vi "Post-Install Custom Action.vi"(10 "Variant":variant) -> (0 "error out":errorcluster)   [LabVIEW 2020]
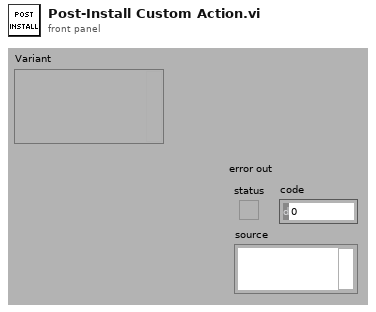
[diagram p1: front panel]
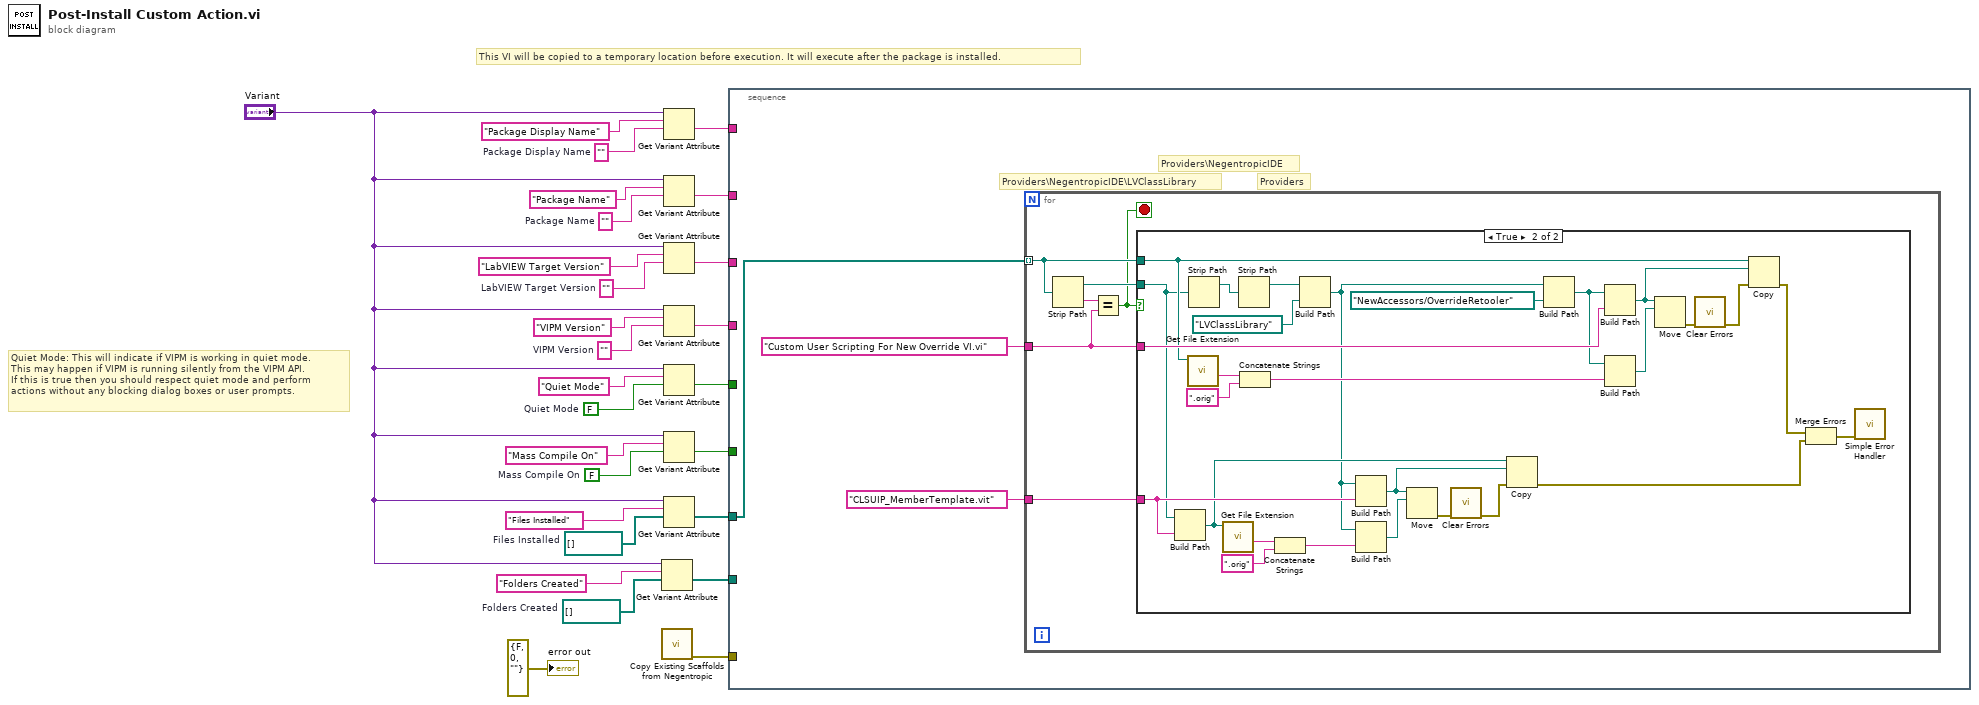
[diagram p0: block diagram]
diagram:
  w2 = path[] []  # Folders Created
  w3 = path[] []  # Files Installed
  w9 = FALSE  # Mass Compile On
  w10 = ""  # Package Display Name
  w17 = FALSE  # Quiet Mode
  w20 = ""  # VIPM Version
  w22 = ""  # LabVIEW Target Version
  w24 = ""  # Package Name
  # "Quiet Mode: This will indicate if VIPM is working in quiet mode.\nThis may happen if VIPM is running silently from the VIPM API.\nIf this is true then you should respect quiet mode and perform\nactions without any blocking dialog boxes or user prompts."
  # "This VI will be copied to a temporary location before execution. It will execute after the package is installed."
  n1 = Get Variant Attribute(Variant="Variant", name="Folders Created", default value (empty Variant)=w2) -> (value=w7:path[])  [unwired: 1 in, 3 out]
  n2 = call "Copy Existing Scaffolds from Negentropic.vi"() -> ("error out"=w1:errorcluster)  [unwired: 11 in]
  n3 = Get Variant Attribute(Variant="Variant", name="Package Display Name", default value (empty Variant)=w10) -> (value=w16:string)  [unwired: 1 in, 3 out]
  n4 = Get Variant Attribute(Variant="Variant", name="Package Name", default value (empty Variant)=w24) -> (value=w15:string)  [unwired: 1 in, 3 out]
  n5 = Get Variant Attribute(Variant="Variant", name="LabVIEW Target Version", default value (empty Variant)=w22) -> (value=w14:string)  [unwired: 1 in, 3 out]
  n6 = Get Variant Attribute(Variant="Variant", name="VIPM Version", default value (empty Variant)=w20) -> (value=w13:string)  [unwired: 1 in, 3 out]
  n7 = Get Variant Attribute(Variant="Variant", name="Quiet Mode", default value (empty Variant)=w17) -> (value=w12:bool)  [unwired: 1 in, 3 out]
  n8 = Get Variant Attribute(Variant="Variant", name="Mass Compile On", default value (empty Variant)=w9) -> (value=w11:bool)  [unwired: 1 in, 3 out]
  n9 = Get Variant Attribute(Variant="Variant", name="Files Installed", default value (empty Variant)=w3) -> (value=w6:path[])  [unwired: 1 in, 3 out]
  n10 = stacked-sequence {
    tunnel: w16 -> [_]
    tunnel: w15 -> [_]
    tunnel: w14 -> [_]
    tunnel: w13 -> [_]
    tunnel: w12 -> [_]
    tunnel: w11 -> [_]
    tunnel: w6 -> [w28]
    tunnel: w7 -> [_]
    tunnel: w1 -> [_]
    frame #0 {
      # "Providers"
      # "Providers\\NegentropicIDE"
      # "Providers\\NegentropicIDE\\LVClassLibrary"
      n11 = for {
        tunnel: w28 -> [w36] mode=indexing
        tunnel: "Custom User Scripting For New Override VI.vi" -> [w31]
        tunnel: "CLSUIP_MemberTemplate.vit" -> [w32]
        stop <- w34 stop-if-true
        n12 = Strip Path(path=w36) -> (stripped path=w35:path, name=w33:string)
        n13 = Equal?(x=w33, y=w31) -> (x = y?=w34:bool)
        n14 = case shown="True" w34 {
          tunnel: w36 -> [_ w60]
          tunnel: w35 -> [_ w43]
          tunnel: w31 -> [_ w61]
          tunnel: w32 -> [_ w50]
          frame False {
          }
          frame True {
            n15 = Build Path(base path=w43, name or relative path=w50) -> (appended path=w48:path)
            n16 = call <vilib>:"Get File Extension.vi"("file"=w60) -> ("filename without extension"=w59:string)  [unwired: 6 in, 4 out]
            n17 = Strip Path(path=w43) -> (stripped path=w64:path)  [unwired: 1 out]
            n18 = call <vilib>:"Get File Extension.vi"("file"=w48) -> ("filename without extension"=w52:string)  [unwired: 6 in, 4 out]
            n19 = Strip Path(path=w64) -> (stripped path=w63:path)  [unwired: 1 out]
            n20 = Concatenate Strings(w59, ".orig" ("string")) -> (w57:string)
            n21 = Concatenate Strings(w52, ".orig" ("string")) -> (w51:string)
            n22 = Build Path(base path=w63, name or relative path=path "LVClassLibrary") -> (appended path=w45:path)
            n23 = Build Path(base path=w45, name or relative path=w50) -> (appended path=w47:path)
            n24 = Build Path(base path=w45, name or relative path=w51) -> (appended path=w49:path)
            n25 = Move(source path=w47, 10:w49) -> (error out=w46:errorcluster)  [unwired: 3 in, 2 out]
            n26 = call <vilib>:"Clear Errors.vi"("error in (no error)"=w46) -> ("error out"=w41:errorcluster)  [unwired: 5 in, 1 out]
            n27 = Copy(8:w41, 10:w47, 11:w48) -> (0:w38:errorcluster)  [unwired: 2 in, 2 out]
            n28 = Build Path(base path=w45, name or relative path=path "NewAccessors/OverrideRetooler") -> (appended path=w42:path)
            n29 = Build Path(base path=w42, name or relative path=w61) -> (appended path=w55:path)
            n30 = Build Path(base path=w42, name or relative path=w57) -> (appended path=w56:path)
            n31 = Move(source path=w55, 10:w56) -> (error out=w54:errorcluster)  [unwired: 3 in, 2 out]
            n32 = call <vilib>:"Clear Errors.vi"("error in (no error)"=w54) -> ("error out"=w40:errorcluster)  [unwired: 5 in, 1 out]
            n33 = Copy(8:w40, 10:w55, 11:w60) -> (0:w39:errorcluster)  [unwired: 2 in, 2 out]
            n34 = Merge Errors(w39, w38) -> (w37:errorcluster)
            n35 = call <vilib>:"Simple Error Handler.vi"("error in (no error)"=w37) -> ()  [unwired: 4 in, 5 out]
          }
        }
      }
    }
  }
  "error out" <- errorcluster {"status"=FALSE, "code"=0, "source"=""} ("error out")
